vi "Convert U64 to I16x4.vi"(7 "U64":u64) -> (8 "4xI16 Array":i16[](array[numeric]))   [LabVIEW 2012]
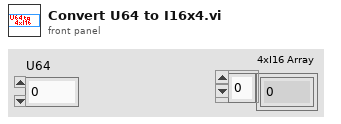
[diagram p1: front panel]
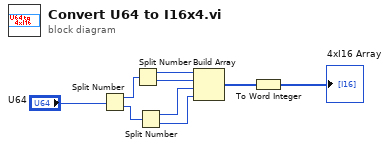
[diagram p0: block diagram]
diagram:
  n1 = Split Number(x="U64") -> (hi(x)=w9:u32, lo(x)=w8:u32)
  n2 = Split Number(x=w9) -> (hi(x)=w6:u16, lo(x)=w5:u16)
  n3 = Split Number(x=w8) -> (hi(x)=w4:u16, lo(x)=w3:u16)
  n4 = Build Array(w6, w5, w4, w3) -> (w2:u16[])
  n5 = To Word Integer(number=w2) -> (16bit integer=→"4xI16 Array":i16[])
